vi "Execute_Table.vi"(1 "Start and Stop Indexes":fxp<+,5,5>) -> (0 "Aborted":bool)   [LabVIEW 2017]
uses:
  <vilib>/rvi/Emulation/niFpgaGetClockAttributes.vi
  <vilib>/rvi/Emulation/niFpgaSctlEmulationGetInTimedLoop.vi
  <vilib>/rvi/Emulation/niFpgaEmulationReportErrorSimple.vi
  <vilib>/rvi/Memory/Memory_Emulation/nirvimemoryFastEmulation.vi
  <vilib>/rvi/Memory/Memory_Emulation/nirvimemoryEmulation.vi
  <vilib>/rvi/Emulation/niFpgaEmulationIsFPGAContextNoSignature.vi
  <vilib>/rvi/DataTransferAndStorage/Container/Common/niFpgaContainerGetUniqueNameForEmu.vi
  <vilib>/rvi/Emulation/niFpgaProcessEmulError.vi
  <vilib>/rvi/errors/nirviReportUnexpectedCaseInternalError (U32).vi
  <vilib>/rvi/Memory/Memory_Emulation/niFpgaMemoryEmulationCacheClearOnFirstRun.vi
  <vilib>/rvi/Memory/Memory_Emulation/nirvimemoryEmulationManagerCache_MakeExclusive.vi
  <vilib>/rvi/Memory/Memory_Emulation/niFpgaMemoryEmulationValidateCache.vi
  <vilib>/rvi/Memory/Memory_Emulation/nirvimemoryEmulationManagerCache_InsertValue.vi
  <vilib>/Utility/error.llb/Clear Errors.vi
  <vilib>/rvi/Memory/Memory_Emulation/nirvimemoryEmulationManagerCache_ReleaseExclusive.vi
  <vilib>/rvi/Memory/Memory_Emulation/nirvimemoryEmulationManagerCache_GetValue.vi
  <vilib>/rvi/Memory/Memory_Emulation/nirvimemoryEmulationManagerCache_SetValue.vi
  <vilib>/rvi/eio/common/nirviEmuTemplateMethod_errors.vi
  <vilib>/rvi/Emulation/niFpgaCriticalErrorInLSC.vi
  <vilib>/rvi/occurrence/nirviWaitOnOccurrenceBase.vi
  <vilib>/rvi/DataTransferAndStorage/Container/XNode/niFpgaContainer.xnode
  <vilib>/rvi/DataTransferAndStorage/Register/Emulation/niFpgaRegisterEmulation.vi
  <vilib>/eio/EIONode/EIONode.xnode
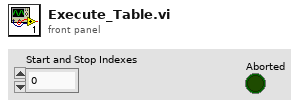
[diagram p1: front panel]
types:
  T1 = cluster{"Boolean array[0]":bool, "Boolean array[1]":bool, "Boolean array[2]":bool, "Boolean array[3]":bool, "Boolean array[4]":bool, "Boolean array[5]":bool, "Boolean array[6]":bool, "Boolean array[7]":bool, "Boolean array[8]":bool, "Boolean array[9]":bool, "Boolean array[10]":bool, "Boolean array[11]":bool, "Boolean array[12]":bool, "Boolean array[13]":bool, "Boolean array[14]":bool, "Boolean array[15]":bool}
  T2 = cluster{"Data":i16, "Data":i16, "Data":i16, "Data":i16}
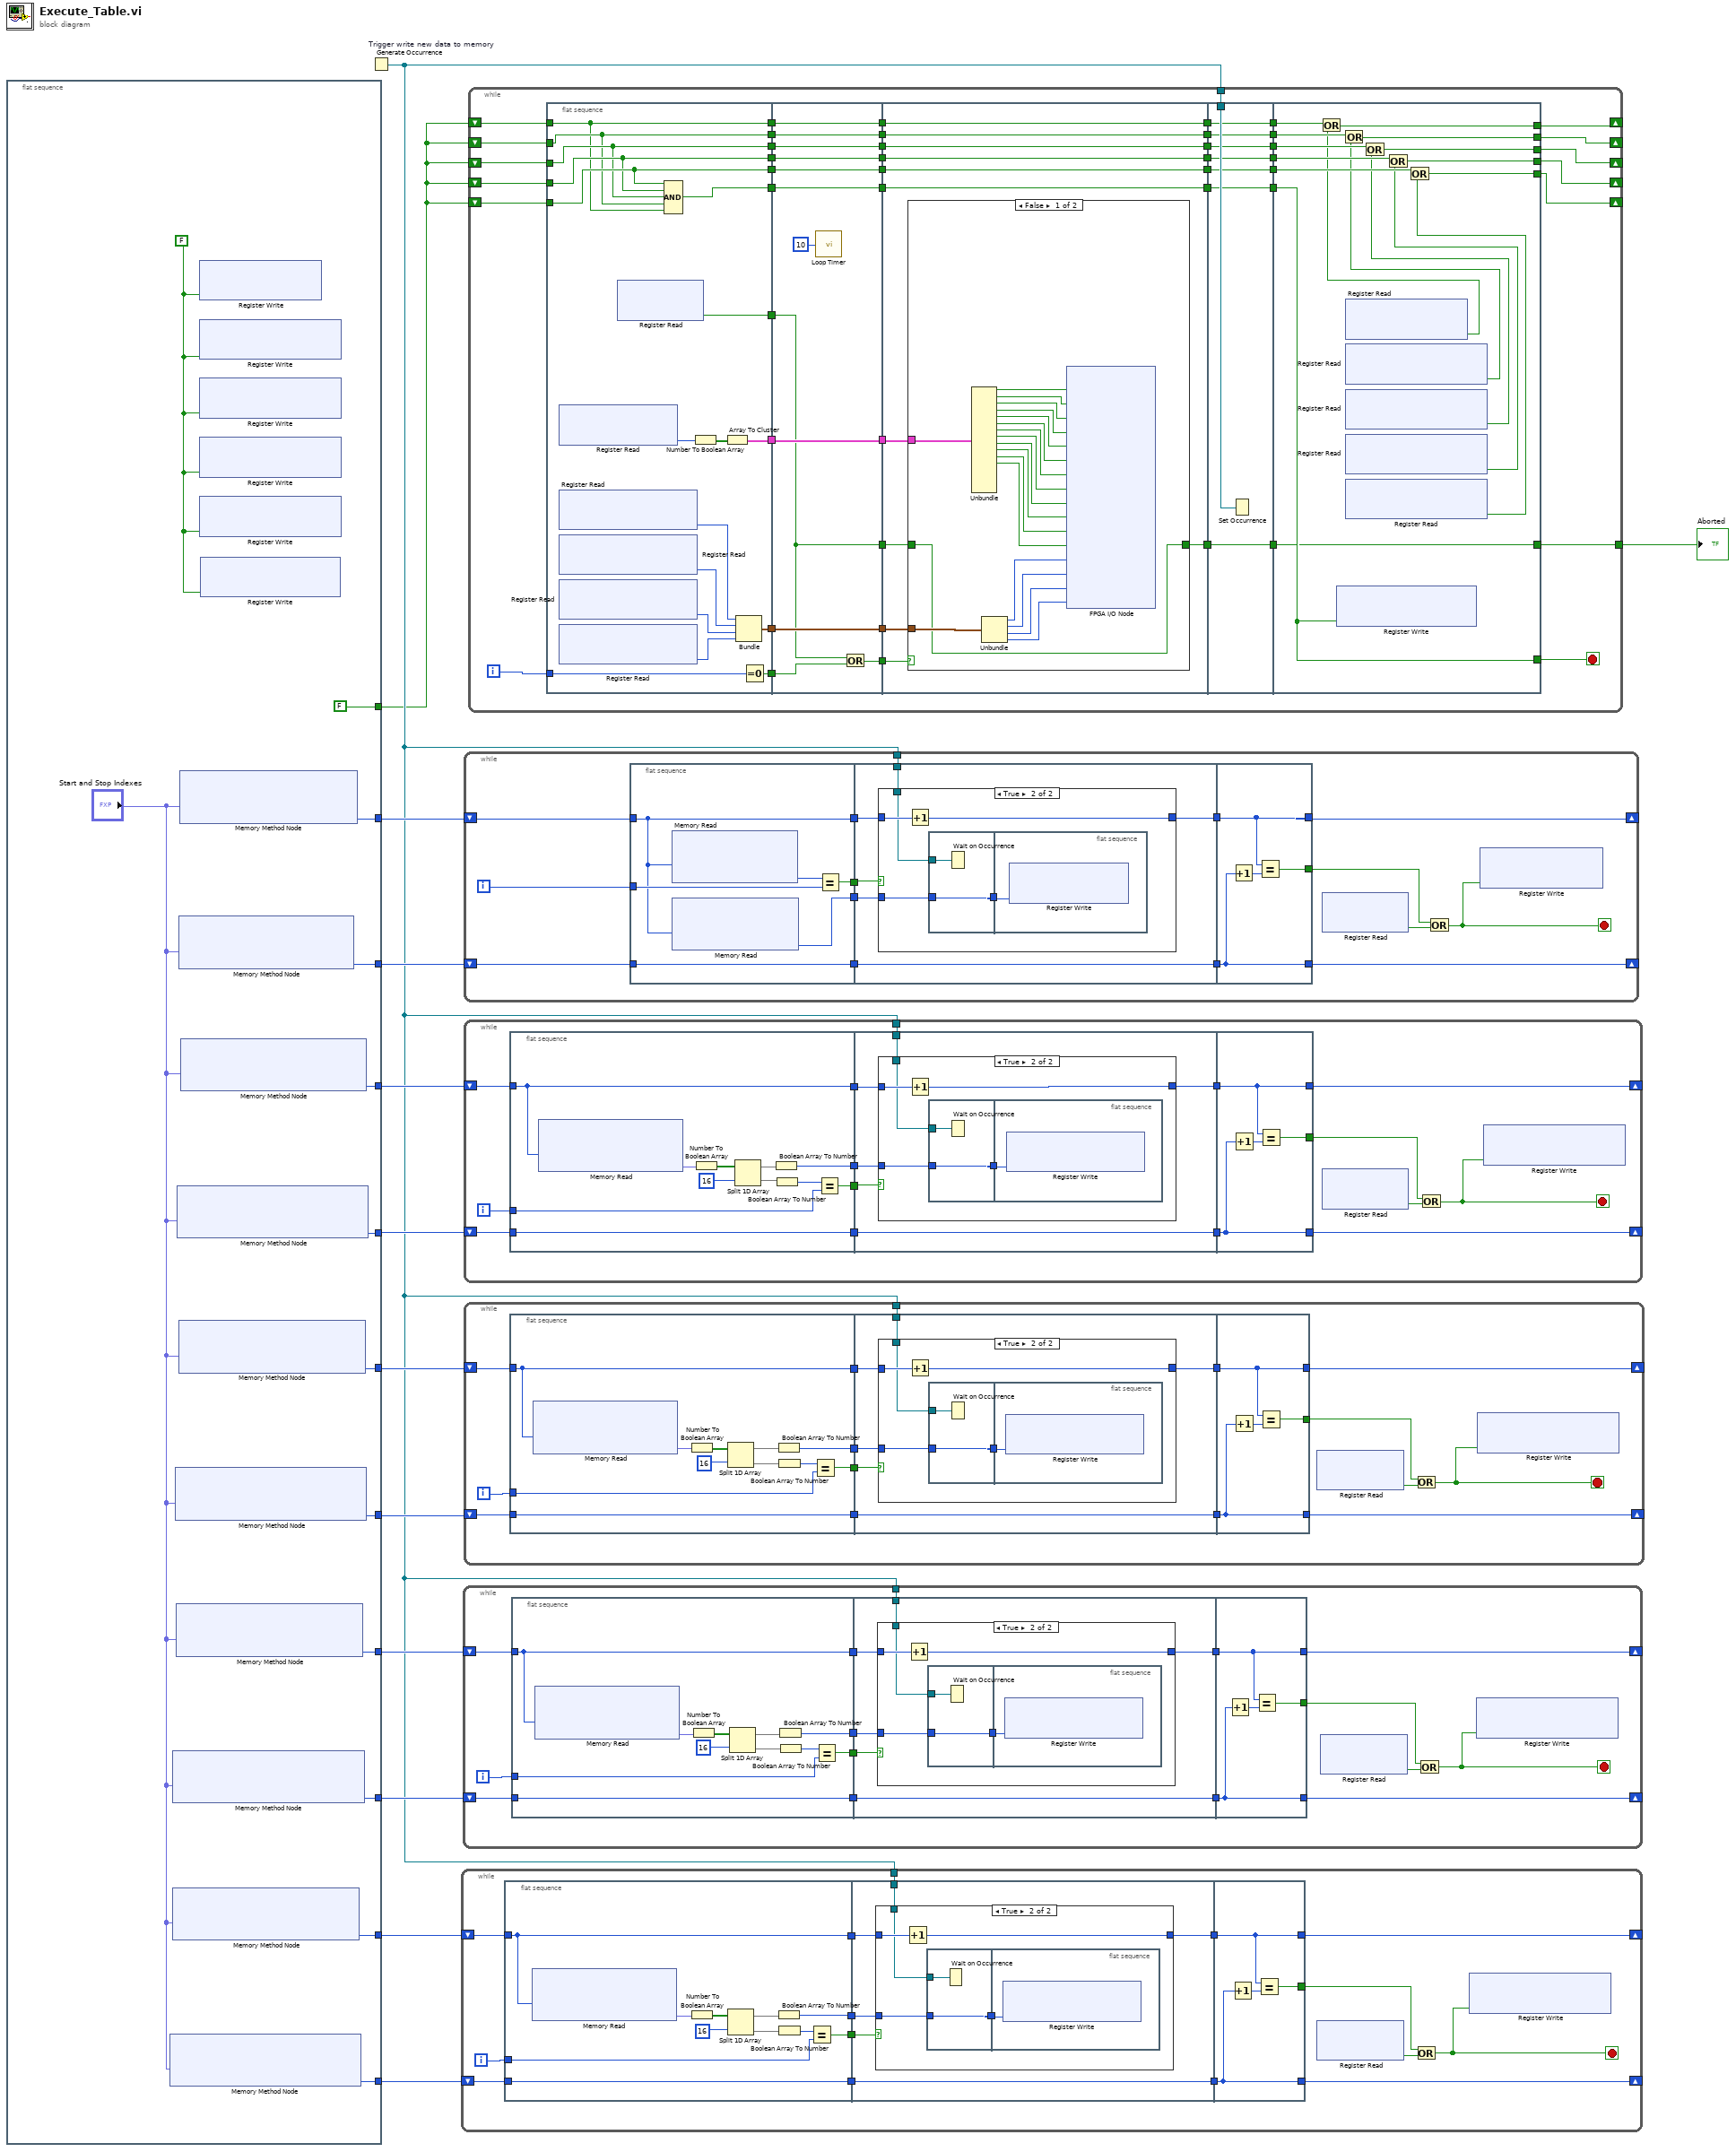
[diagram p0: block diagram]
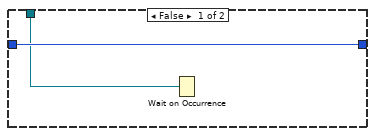
[diagram p2: hidden frame]
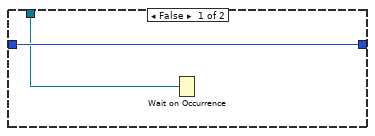
[diagram p3: hidden frame]
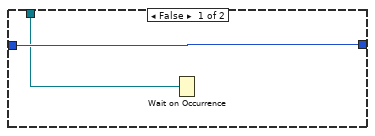
[diagram p4: hidden frame]
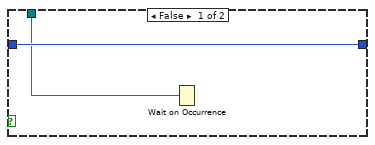
[diagram p5: hidden frame]
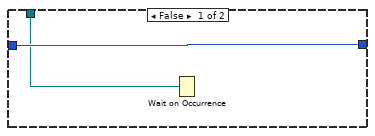
[diagram p6: hidden frame]
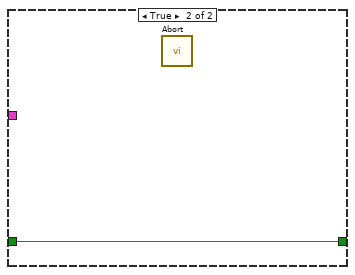
[diagram p7: hidden frame]
diagram:
  n1 = flat-sequence {
    tunnel: [w26] -> w13
    tunnel: [w25] -> w12
    tunnel: [w24] -> w11
    tunnel: [w23] -> w10
    tunnel: [w22] -> w9
    tunnel: [w21] -> w8
    tunnel: [w20] -> w7
    tunnel: [w19] -> w6
    tunnel: [w18] -> w5
    tunnel: [w17] -> w4
    tunnel: [FALSE] -> w1
    frame #0 {
      w15 = FALSE ("Data")
      n2 = xnode ("Memory Method Node")("Address"="Start and Stop Indexes") -> ("Data"=w17:u16)  [unwired: 1 in, 1 out]
      n3 = xnode ("Memory Method Node")("Address"="Start and Stop Indexes") -> ("Data"=w19:u16)  [unwired: 1 in, 1 out]
      n4 = xnode ("Memory Method Node")("Address"="Start and Stop Indexes") -> ("Data"=w18:u16)  [unwired: 1 in, 1 out]
      n5 = xnode ("Memory Method Node")("Address"="Start and Stop Indexes") -> ("Data"=w21:u16)  [unwired: 1 in, 1 out]
      n6 = xnode ("Memory Method Node")("Address"="Start and Stop Indexes") -> ("Data"=w20:u16)  [unwired: 1 in, 1 out]
      n7 = xnode ("Memory Method Node")("Address"="Start and Stop Indexes") -> ("Data"=w24:u16)  [unwired: 1 in, 1 out]
      n8 = xnode ("Memory Method Node")("Address"="Start and Stop Indexes") -> ("Data"=w25:u16)  [unwired: 1 in, 1 out]
      n9 = xnode ("Memory Method Node")("Address"="Start and Stop Indexes") -> ("Data"=w22:u16)  [unwired: 1 in, 1 out]
      n10 = xnode ("Memory Method Node")("Address"="Start and Stop Indexes") -> ("Data"=w26:u16)  [unwired: 1 in, 1 out]
      n11 = xnode ("Memory Method Node")("Address"="Start and Stop Indexes") -> ("Data"=w23:u16)  [unwired: 1 in, 1 out]
      n12 = xnode ("Register Write")("Data"=w15) -> ()  [unwired: 1 in, 1 out]
      n13 = xnode ("Register Write")("Data"=w15) -> ()  [unwired: 1 in, 1 out]
      n14 = xnode ("Register Write")("Data"=w15) -> ()  [unwired: 1 in, 1 out]
      n15 = xnode ("Register Write")("Data"=w15) -> ()  [unwired: 1 in, 1 out]
      n16 = xnode ("Register Write")("Data"=w15) -> ()  [unwired: 1 in, 1 out]
      n17 = xnode ("Register Write")("Data"=w15) -> ()  [unwired: 1 in, 1 out]
    }
  }
  n18 = Generate Occurrence "Trigger write new data to memory"() -> (w3:refnum<k4>)
  n19 = while {
    tunnel: w3 -> [w31]
    shift-right: [w30] -> _
    shift-left: w5 -> [w32]
    shift-right: [w28] -> _
    shift-left: w4 -> [w34]
    i -> [w41]
    stop <- w29 stop-if-true
    n20 = flat-sequence {
      tunnel: w41 -> [w46]
      tunnel: [w48] -> w40
      tunnel: [w42] -> w39
      tunnel: [w44] -> w38
      tunnel: [w45] -> w35
      tunnel: w34 -> [w45]
      tunnel: w32 -> [w44]
      tunnel: w40 -> [w56]
      tunnel: w39 -> [w58]
      tunnel: w38 -> [w57]
      tunnel: [w55] -> w37
      tunnel: [w54] -> w36
      tunnel: w35 -> [w54]
      tunnel: w31 -> [w53]
      tunnel: [w71] -> w30
      tunnel: [w70] -> w27
      tunnel: w36 -> [w69]
      tunnel: w37 -> [w71]
      tunnel: [w69] -> w28
      frame #0 {
        n21 = xnode ("Memory Read")("Address"=w44) -> ("Data"=w52:fxp<+/-,48,48>)  [unwired: 1 in, 1 out]
        n22 = Number To Boolean Array(number=w52) -> (Boolean array=w51:bool[])
        n23 = Split 1D Array(array=w51, index=16) -> (first subarray=w49:bool[], second subarray=w47:bool[])
        n24 = Boolean Array To Number(Boolean array=w49) -> (number=w42:i16)
        n25 = Boolean Array To Number(Boolean array=w47) -> (number=w43:u32)
        n26 = Equal?(x=w43, y=w46) -> (x = y?=w48:bool)
      }
      frame #1 {
        n27 = case shown="True" w56 {
          tunnel: w57 -> [w60 w65]
          tunnel: [w60 w64] -> w55
          tunnel: w58 -> [_ w62]
          tunnel: w53 -> [w59 w61]
          frame False {
            n28 = Wait on Occurrence(2:w59) -> ()  [unwired: 2 in, 1 out]
          }
          frame True {
            n29 = Increment(x=w65) -> (x+1=w64:u16)
            n30 = flat-sequence {
              tunnel: w61 -> [w67]
              tunnel: [w66] -> w63
              tunnel: w62 -> [w66]
              tunnel: w63 -> [w68]
              frame #0 {
                n31 = Wait on Occurrence(2:w67) -> ()  [unwired: 2 in, 1 out]
              }
              frame #1 {
                n32 = xnode ("Register Write")("Data"=w68) -> ()  [unwired: 1 in, 1 out]
              }
            }
          }
        }
      }
      frame #2 {
        n33 = Increment(x=w69) -> (x+1=w72:u16)
        n34 = Equal?(x=w71, y=w72) -> (x = y?=w70:bool)
      }
    }
    n35 = xnode ("Register Read")() -> ("Data"=w33:bool)  [unwired: 1 in, 1 out]
    n36 = Or(x=w27, y=w33) -> (x .or. y?=w29:bool)
    n37 = xnode ("Register Write")("Data"=w29) -> ()  [unwired: 1 in, 1 out]
  }
  n38 = while {
    tunnel: w3 -> [w77]
    shift-right: [w76] -> _
    shift-left: w7 -> [w78]
    shift-right: [w74] -> _
    shift-left: w6 -> [w80]
    i -> [w87]
    stop <- w75 stop-if-true
    n39 = flat-sequence {
      tunnel: w87 -> [w92]
      tunnel: [w94] -> w86
      tunnel: [w89] -> w85
      tunnel: [w90] -> w84
      tunnel: [w91] -> w81
      tunnel: w80 -> [w91]
      tunnel: w78 -> [w90]
      tunnel: w86 -> [w102]
      tunnel: w85 -> [w104]
      tunnel: w84 -> [w103]
      tunnel: [w101] -> w83
      tunnel: [w100] -> w82
      tunnel: w81 -> [w100]
      tunnel: w77 -> [w99]
      tunnel: [w117] -> w76
      tunnel: [w116] -> w73
      tunnel: w82 -> [w115]
      tunnel: w83 -> [w117]
      tunnel: [w115] -> w74
      frame #0 {
        n40 = xnode ("Memory Read")("Address"=w90) -> ("Data"=w98:fxp<+,48,48>)  [unwired: 1 in, 1 out]
        n41 = Number To Boolean Array(number=w98) -> (Boolean array=w97:bool[])
        n42 = Split 1D Array(array=w97, index=16) -> (first subarray=w95:bool[], second subarray=w93:bool[])
        n43 = Boolean Array To Number(Boolean array=w95) -> (number=w89:i16)
        n44 = Boolean Array To Number(Boolean array=w93) -> (number=w88:u32)
        n45 = Equal?(x=w88, y=w92) -> (x = y?=w94:bool)
      }
      frame #1 {
        n46 = case shown="True" w102 {
          tunnel: w103 -> [w106 w111]
          tunnel: [w106 w110] -> w101
          tunnel: w104 -> [_ w108]
          tunnel: w99 -> [w105 w107]
          frame False {
            n47 = Wait on Occurrence(2:w105) -> ()  [unwired: 2 in, 1 out]
          }
          frame True {
            n48 = Increment(x=w111) -> (x+1=w110:u16)
            n49 = flat-sequence {
              tunnel: w107 -> [w113]
              tunnel: [w112] -> w109
              tunnel: w108 -> [w112]
              tunnel: w109 -> [w114]
              frame #0 {
                n50 = Wait on Occurrence(2:w113) -> ()  [unwired: 2 in, 1 out]
              }
              frame #1 {
                n51 = xnode ("Register Write")("Data"=w114) -> ()  [unwired: 1 in, 1 out]
              }
            }
          }
        }
      }
      frame #2 {
        n52 = Increment(x=w115) -> (x+1=w118:u16)
        n53 = Equal?(x=w117, y=w118) -> (x = y?=w116:bool)
      }
    }
    n54 = xnode ("Register Read")() -> ("Data"=w79:bool)  [unwired: 1 in, 1 out]
    n55 = Or(x=w73, y=w79) -> (x .or. y?=w75:bool)
    n56 = xnode ("Register Write")("Data"=w75) -> ()  [unwired: 1 in, 1 out]
  }
  n57 = while {
    shift-right: [w129] -> _
    shift-left: w13 -> [w128]
    tunnel: w3 -> [w121]
    shift-right: [w119] -> _
    shift-left: w12 -> [w124]
    i -> [w133]
    stop <- w120 stop-if-true
    n58 = flat-sequence {
      tunnel: w128 -> [w135]
      tunnel: w133 -> [w138]
      tunnel: [w139] -> w132
      tunnel: [w134] -> w131
      tunnel: [w135] -> w130
      tunnel: [w137] -> w125
      tunnel: w124 -> [w137]
      tunnel: w132 -> [w143]
      tunnel: w131 -> [w145]
      tunnel: w130 -> [w144]
      tunnel: [w142] -> w127
      tunnel: [w141] -> w126
      tunnel: w125 -> [w141]
      tunnel: w121 -> [w140]
      tunnel: [w158] -> w129
      tunnel: [w157] -> w123
      tunnel: w126 -> [w156]
      tunnel: w127 -> [w158]
      tunnel: [w156] -> w119
      frame #0 {
        n59 = xnode ("Memory Read")("Address"=w135) -> ("Data"=w136:u32)  [unwired: 1 in, 1 out]
        n60 = xnode ("Memory Read")("Address"=w135) -> ("Data"=w134:u16)  [unwired: 1 in, 1 out]
        n61 = Equal?(x=w136, y=w138) -> (x = y?=w139:bool)
      }
      frame #1 {
        n62 = case shown="True" w143 {
          tunnel: w144 -> [w147 w152]
          tunnel: [w147 w151] -> w142
          tunnel: w145 -> [_ w149]
          tunnel: w140 -> [w146 w148]
          frame False {
            n63 = Wait on Occurrence(2:w146) -> ()  [unwired: 2 in, 1 out]
          }
          frame True {
            n64 = Increment(x=w152) -> (x+1=w151:u16)
            n65 = flat-sequence {
              tunnel: [w154] -> w150
              tunnel: w149 -> [w154]
              tunnel: w148 -> [w153]
              tunnel: w150 -> [w155]
              frame #0 {
                n66 = Wait on Occurrence(2:w153) -> ()  [unwired: 2 in, 1 out]
              }
              frame #1 {
                n67 = xnode ("Register Write")("Data"=w155) -> ()  [unwired: 1 in, 1 out]
              }
            }
          }
        }
      }
      frame #2 {
        n68 = Increment(x=w156) -> (x+1=w159:u16)
        n69 = Equal?(x=w158, y=w159) -> (x = y?=w157:bool)
      }
    }
    n70 = xnode ("Register Read")() -> ("Data"=w122:bool)  [unwired: 1 in, 1 out]
    n71 = Or(x=w123, y=w122) -> (x .or. y?=w120:bool)
    n72 = xnode ("Register Write")("Data"=w120) -> ()  [unwired: 1 in, 1 out]
  }
  n73 = while {
    tunnel: w3 -> [w163]
    shift-right: [w162] -> _
    shift-left: w10 -> [w164]
    shift-right: [w160] -> _
    shift-left: w11 -> [w167]
    i -> [w174]
    stop <- w161 stop-if-true
    n74 = flat-sequence {
      tunnel: w174 -> [w180]
      tunnel: [w182] -> w173
      tunnel: [w175] -> w172
      tunnel: [w178] -> w171
      tunnel: [w179] -> w168
      tunnel: w167 -> [w179]
      tunnel: w164 -> [w178]
      tunnel: w173 -> [w189]
      tunnel: w172 -> [w191]
      tunnel: w171 -> [w190]
      tunnel: [w188] -> w170
      tunnel: [w187] -> w169
      tunnel: w168 -> [w187]
      tunnel: w163 -> [w186]
      tunnel: [w204] -> w162
      tunnel: [w203] -> w166
      tunnel: w169 -> [w202]
      tunnel: w170 -> [w204]
      tunnel: [w202] -> w160
      frame #0 {
        n75 = xnode ("Memory Read")("Address"=w178) -> ("Data"=w185:fxp<+,48,48>)  [unwired: 1 in, 1 out]
        n76 = Number To Boolean Array(number=w185) -> (Boolean array=w177:bool[])
        n77 = Split 1D Array(array=w177, index=16) -> (first subarray=w183:bool[], second subarray=w181:bool[])
        n78 = Boolean Array To Number(Boolean array=w183) -> (number=w175:i16)
        n79 = Boolean Array To Number(Boolean array=w181) -> (number=w176:u32)
        n80 = Equal?(x=w176, y=w180) -> (x = y?=w182:bool)
      }
      frame #1 {
        n81 = case shown="True" w189 {
          tunnel: w190 -> [w193 w198]
          tunnel: [w193 w197] -> w188
          tunnel: w191 -> [_ w195]
          tunnel: w186 -> [w192 w194]
          frame False {
            n82 = Wait on Occurrence(2:w192) -> ()  [unwired: 2 in, 1 out]
          }
          frame True {
            n83 = Increment(x=w198) -> (x+1=w197:u16)
            n84 = flat-sequence {
              tunnel: w194 -> [w200]
              tunnel: [w199] -> w196
              tunnel: w195 -> [w199]
              tunnel: w196 -> [w201]
              frame #0 {
                n85 = Wait on Occurrence(2:w200) -> ()  [unwired: 2 in, 1 out]
              }
              frame #1 {
                n86 = xnode ("Register Write")("Data"=w201) -> ()  [unwired: 1 in, 1 out]
              }
            }
          }
        }
      }
      frame #2 {
        n87 = Increment(x=w202) -> (x+1=w205:u16)
        n88 = Equal?(x=w204, y=w205) -> (x = y?=w203:bool)
      }
    }
    n89 = xnode ("Register Read")() -> ("Data"=w165:bool)  [unwired: 1 in, 1 out]
    n90 = Or(x=w166, y=w165) -> (x .or. y?=w161:bool)
    n91 = xnode ("Register Write")("Data"=w161) -> ()  [unwired: 1 in, 1 out]
  }
  n92 = while {
    tunnel: w3 -> [w210]
    shift-right: [w209] -> _
    shift-left: w9 -> [w211]
    shift-right: [w207] -> _
    shift-left: w8 -> [w214]
    i -> [w220]
    stop <- w208 stop-if-true
    n93 = flat-sequence {
      tunnel: w220 -> [w225]
      tunnel: [w227] -> w219
      tunnel: [w223] -> w218
      tunnel: [w224] -> w215
      tunnel: w214 -> [w224]
      tunnel: w211 -> [w223]
      tunnel: [w222] -> w206
      tunnel: w219 -> [w235]
      tunnel: w218 -> [w236]
      tunnel: [w234] -> w217
      tunnel: [w233] -> w216
      tunnel: w215 -> [w233]
      tunnel: w210 -> [w232]
      tunnel: w206 -> [w237]
      tunnel: [w250] -> w209
      tunnel: [w249] -> w213
      tunnel: w216 -> [w248]
      tunnel: w217 -> [w250]
      tunnel: [w248] -> w207
      frame #0 {
        n94 = xnode ("Memory Read")("Address"=w223) -> ("Data"=w231:fxp<+,48,48>)  [unwired: 1 in, 1 out]
        n95 = Number To Boolean Array(number=w231) -> (Boolean array=w230:bool[])
        n96 = Split 1D Array(array=w230, index=16) -> (first subarray=w228:bool[], second subarray=w226:bool[])
        n97 = Boolean Array To Number(Boolean array=w228) -> (number=w222:i16)
        n98 = Boolean Array To Number(Boolean array=w226) -> (number=w221:u32)
        n99 = Equal?(x=w221, y=w225) -> (x = y?=w227:bool)
      }
      frame #1 {
        n100 = case shown="True" w235 {
          tunnel: w236 -> [w239 w244]
          tunnel: [w239 w243] -> w234
          tunnel: w237 -> [_ w241]
          tunnel: w232 -> [w238 w240]
          frame False {
            n101 = Wait on Occurrence(2:w238) -> ()  [unwired: 2 in, 1 out]
          }
          frame True {
            n102 = Increment(x=w244) -> (x+1=w243:u16)
            n103 = flat-sequence {
              tunnel: w240 -> [w246]
              tunnel: [w245] -> w242
              tunnel: w241 -> [w245]
              tunnel: w242 -> [w247]
              frame #0 {
                n104 = Wait on Occurrence(2:w246) -> ()  [unwired: 2 in, 1 out]
              }
              frame #1 {
                n105 = xnode ("Register Write")("Data"=w247) -> ()  [unwired: 1 in, 1 out]
              }
            }
          }
        }
      }
      frame #2 {
        n106 = Increment(x=w248) -> (x+1=w251:u16)
        n107 = Equal?(x=w250, y=w251) -> (x = y?=w249:bool)
      }
    }
    n108 = xnode ("Register Read")() -> ("Data"=w212:bool)  [unwired: 1 in, 1 out]
    n109 = Or(x=w213, y=w212) -> (x .or. y?=w208:bool)
    n110 = xnode ("Register Write")("Data"=w208) -> ()  [unwired: 1 in, 1 out]
  }
  n111 = while {
    tunnel: w3 -> [w297]
    shift-right: [w262] -> _
    shift-left: w1 -> [w292]
    shift-right: [w261] -> _
    shift-left: w1 -> [w287]
    shift-right: [w260] -> _
    shift-left: w1 -> [w282]
    shift-right: [w259] -> _
    shift-left: w1 -> [w277]
    shift-right: [w258] -> _
    shift-left: w1 -> [w272]
    tunnel: [w255] -> w2
    i -> [w252]
    stop <- w271 stop-if-true
    n112 = flat-sequence {
      tunnel: w252 -> [w300]
      tunnel: [w315] -> w298
      tunnel: [w310] -> w293
      tunnel: w292 -> [w310]
      tunnel: [w311] -> w288
      tunnel: w287 -> [w311]
      tunnel: [w312] -> w283
      tunnel: w282 -> [w312]
      tunnel: [w313] -> w278
      tunnel: w277 -> [w313]
      tunnel: [w314] -> w273
      tunnel: w272 -> [w314]
      tunnel: [w302] -> w267
      tunnel: [w305] -> w265
      tunnel: [w303] -> w264
      tunnel: [w301] -> w257
      tunnel: [w319] -> w299
      tunnel: w298 -> [w327]
      tunnel: [w326] -> w294
      tunnel: w293 -> [w326]
      tunnel: [w325] -> w289
      tunnel: w288 -> [w325]
      tunnel: [w324] -> w284
      tunnel: w283 -> [w324]
      tunnel: [w323] -> w279
      tunnel: w278 -> [w323]
      tunnel: [w322] -> w274
      tunnel: w273 -> [w322]
      tunnel: [w318] -> w268
      tunnel: w267 -> [w318]
      tunnel: [w321] -> w266
      tunnel: w265 -> [w321]
      tunnel: w264 -> [w320]
      tunnel: [w320] -> w263
      tunnel: w257 -> [w317]
      tunnel: [w317] -> w256
      tunnel: w299 -> [w339]
      tunnel: [w338] -> w295
      tunnel: w294 -> [w338]
      tunnel: [w337] -> w290
      tunnel: w289 -> [w337]
      tunnel: [w336] -> w285
      tunnel: w284 -> [w336]
      tunnel: [w335] -> w280
      tunnel: w279 -> [w335]
      tunnel: [w334] -> w275
      tunnel: w274 -> [w334]
      tunnel: [w333] -> w269
      tunnel: w268 -> [w333]
      tunnel: w266 -> [w332]
      tunnel: w263 -> [w331]
      tunnel: w256 -> [w330]
      tunnel: [w329] -> w253
      tunnel: w297 -> [w367]
      tunnel: [w366] -> w296
      tunnel: w295 -> [w366]
      tunnel: [w365] -> w291
      tunnel: w290 -> [w365]
      tunnel: [w364] -> w286
      tunnel: w285 -> [w364]
      tunnel: [w363] -> w281
      tunnel: w280 -> [w363]
      tunnel: [w362] -> w276
      tunnel: w275 -> [w362]
      tunnel: [w361] -> w270
      tunnel: w269 -> [w361]
      tunnel: [w360] -> w254
      tunnel: w253 -> [w360]
      tunnel: w296 -> [w383]
      tunnel: [w384] -> w262
      tunnel: w291 -> [w382]
      tunnel: [w381] -> w261
      tunnel: [w378] -> w260
      tunnel: w286 -> [w380]
      tunnel: w281 -> [w379]
      tunnel: [w377] -> w259
      tunnel: w276 -> [w376]
      tunnel: [w375] -> w258
      tunnel: [w369] -> w271
      tunnel: w270 -> [w369]
      tunnel: [w368] -> w255
      tunnel: w254 -> [w368]
      frame #0 {
        n113 = xnode ("Register Read")() -> ("Data"=w316:u16)  [unwired: 1 in, 1 out]
        n114 = xnode ("Register Read")() -> ("Data"=w309:i16)  [unwired: 1 in, 1 out]
        n115 = xnode ("Register Read")() -> ("Data"=w308:i16)  [unwired: 1 in, 1 out]
        n116 = xnode ("Register Read")() -> ("Data"=w307:i16)  [unwired: 1 in, 1 out]
        n117 = xnode ("Register Read")() -> ("Data"=w306:i16)  [unwired: 1 in, 1 out]
        n118 = xnode ("Register Read")() -> ("Data"=w301:bool)  [unwired: 1 in, 1 out]
        n119 = Compound Arithmetic op=AND(w314, w313, w312, w311, w310) -> (w302:bool)
        n120 = Number To Boolean Array(number=w316) -> (Boolean array=w304:bool[])
        n121 = Array To Cluster(array=w304) -> (cluster=w303:T1)
        n122 = Bundle("Data"=w309, "Data"=w308, "Data"=w307, "Data"=w306) -> (w305:T2)  [unwired: 1 in]
        n123 = Equal To 0?(x=w300) -> (x = 0?=w315:bool)
      }
      frame #1 {
        n124 = call "Loop Timer"("Count(uSec)"=u8 10) -> ()  [unwired: 1 out]
        n125 = Or(x=w317, y=w327) -> (x .or. y?=w319:bool)
      }
      frame #2 {
        n126 = case shown="False" w339 {
          tunnel: w332 -> [w358 _]
          tunnel: w331 -> [w341 _]
          tunnel: w330 -> [w340 w359]
          tunnel: [w340 w359] -> w329
          frame False {
            n127 = Unbundle(w341) -> ("Boolean array[0]"=w342:bool, "Boolean array[1]"=w343:bool, "Boolean array[2]"=w353:bool, "Boolean array[3]"=w352:bool, "Boolean array[4]"=w351:bool, "Boolean array[5]"=w350:bool, "Boolean array[6]"=w349:bool, "Boolean array[7]"=w348:bool, "Boolean array[8]"=w347:bool, "Boolean array[9]"=w346:bool, "Boolean array[10]"=w345:bool, "Boolean array[11]"=w344:bool)  [unwired: 4 out]
            n128 = Unbundle(w358) -> ("Data"=w357:i16, "Data"=w356:i16, "Data"=w355:i16, "Data"=w354:i16)
            n129 = xnode "FPGA I/O Node"("Mod2/DIO0"=w342, "Mod2/DIO1"=w343, "Mod2/DIO2"=w353, "Mod2/DIO3"=w352, "Mod3/DIO0"=w351, "Mod3/DIO1"=w350, "Mod3/DIO2"=w349, "Mod3/DIO3"=w348, "Mod4/DIO0"=w347, "Mod4/DIO1"=w346, "Mod4/DIO2"=w345, "Mod4/DIO3"=w344, "Z Stage"=w357, "Mod1/AO1"=w356, "Mod1/AO2"=w355, "Mod1/AO3"=w354) -> ()  [unwired: 16 in, 16 out]
          }
          frame True {
            n130 = call "Abort.vi"() -> ()  [unwired: 12 in]
          }
        }
      }
      frame #3 {
        n131 = Set Occurrence(w367) -> ()
      }
      frame #4 {
        n132 = xnode ("Register Write")("Data"=w369) -> ()  [unwired: 1 in, 1 out]
        n133 = xnode ("Register Read")() -> ("Data"=w374:bool)  [unwired: 1 in, 1 out]
        n134 = Or(x=w383, y=w374) -> (x .or. y?=w384:bool)
        n135 = xnode ("Register Read")() -> ("Data"=w373:bool)  [unwired: 1 in, 1 out]
        n136 = Or(x=w382, y=w373) -> (x .or. y?=w381:bool)
        n137 = xnode ("Register Read")() -> ("Data"=w372:bool)  [unwired: 1 in, 1 out]
        n138 = xnode ("Register Read")() -> ("Data"=w371:bool)  [unwired: 1 in, 1 out]
        n139 = xnode ("Register Read")() -> ("Data"=w370:bool)  [unwired: 1 in, 1 out]
        n140 = Or(x=w380, y=w372) -> (x .or. y?=w378:bool)
        n141 = Or(x=w379, y=w371) -> (x .or. y?=w377:bool)
        n142 = Or(x=w376, y=w370) -> (x .or. y?=w375:bool)
      }
    }
  }
  "Aborted" <- w2
